vi "Add Case Structure Frame (by Name).vi"(8 "error in (no error)":errorcluster, 10 "Frame name":string, 11 "CaseStructure in":refnum<vi>) -> (0 "error out":errorcluster, 2 "Case Frame":refnum<vi>, 3 "CaseStructure out":refnum<vi>)   [LabVIEW 2019, in "gRPC Template Creation Utility.lvlib"]
uses:
  gRPC Template Creation Utility.lvlib
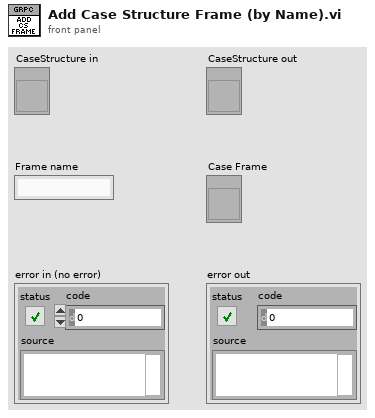
[diagram p1: front panel]
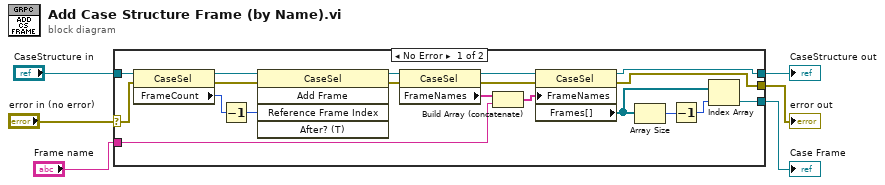
[diagram p0: block diagram]
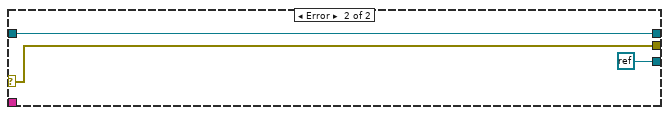
[diagram p2: hidden frame]
diagram:
  n1 = case shown="No Error" "error in (no error)" {
    selector: "error in (no error)" -> [w15 w28]
    tunnel: [w16 w27] -> w6
    tunnel: [w11 w28] -> w5
    tunnel: "CaseStructure in" -> [w20 w27]
    tunnel: "Frame name" -> [w21 _]
    tunnel: [w7 refnum<k0> refnum] -> w1
    frame No Error {
      n2 = property class="CaseSel"(reference=w20, error in=w15) -> (reference out=w19:refnum<vi>, error out=w14:errorcluster, "FrameCount"=w25:i32)
      n3 = Decrement(x=w25) -> (x-1=w24:i32)
      n4 = invoke class="CaseSel" method="Add Frame"(reference=w19, error in=w14, "Reference Frame Index"=w24) -> (reference out=w18:refnum<vi>, error out=w13:errorcluster)  [unwired: 2 in, 3 out]
      n5 = property class="CaseSel"(reference=w18, error in=w13) -> (reference out=w17:refnum<vi>, error out=w12:errorcluster, "FrameNames"=w23:string[])
      n6 = Build Array (concatenate)(w23, w21) -> (w22:string[])
      n7 = property class="CaseSel"(reference=w17, error in=w12, "FrameNames"=w22) -> (reference out=w16:refnum<vi>, error out=w11:errorcluster, "Frames[]"=w10:refnum<vi>[])
      n8 = Array Size(array=w10) -> (size(s)=w8:i32)
      n9 = Decrement(x=w8) -> (x-1=w9:i32)
      n10 = Index Array(array=w10, index=w9) -> (element=w7:refnum<vi>)
    }
    frame Error {
    }
  }
  "error out" <- w5
  "CaseStructure out" <- w6
  "Case Frame" <- w1
